vi "RP100output.vi"(8 "错误输入（无错误）":errorcluster, 11 "VISA资源名称":refnum<visa-resource-name>) -> (0 "错误输出":errorcluster, 1 "OUTPUT 2":dbl, 2 "OUTPUT 1":dbl, 3 "VISA资源名称输出":refnum<visa-resource-name>)   [LabVIEW 2019, in "RP100.lvlib"]
uses:
  RP100.lvlib
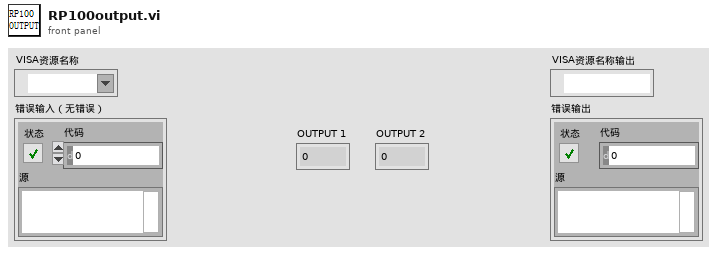
[diagram p1: front panel]
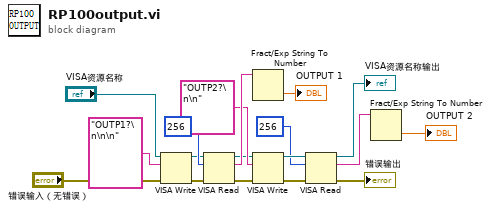
[diagram p0: block diagram]
diagram:
  n1 = VISA Write(VISA resource name="VISA资源名称", write buffer="OUTP1?\n\n\n" ("写入缓冲区"), error in (no error)="错误输入（无错误）") -> (VISA resource name out=w11:refnum<visa-resource-name>, error out=w10:errorcluster)  [unwired: 1 out]
  n2 = VISA Read(VISA resource name=w11, byte count=u32 256 ("字节总数"), error in (no error)=w10) -> (VISA resource name out=w9:refnum<visa-resource-name>, read buffer=w14:string, error out=w8:errorcluster)  [unwired: 1 out]
  n3 = Fract/Exp String To Number(string=w14) -> (number=→"OUTPUT 1":dbl)  [unwired: 3 in, 1 out]
  n4 = VISA Write(VISA resource name=w9, write buffer="OUTP2?\n\n" ("写入缓冲区"), error in (no error)=w8) -> (VISA resource name out=w7:refnum<visa-resource-name>, error out=w6:errorcluster)  [unwired: 1 out]
  n5 = VISA Read(VISA resource name=w7, byte count=u32 256 ("字节总数"), error in (no error)=w6) -> (VISA resource name out=→"VISA资源名称输出":refnum<visa-resource-name>, read buffer=w1:string, error out=→"错误输出":errorcluster)  [unwired: 1 out]
  n6 = Fract/Exp String To Number(string=w1) -> (number=→"OUTPUT 2":dbl)  [unwired: 3 in, 1 out]
